vi "CSC_QuadPlannerAdv.vi"(5 "TorqueRelativeWeight":dbl[](array[numeric]), 6 "F range":cluster{"Fmin":dbl, "Fmax":dbl}, 7 "Weight(1e-6)":dbl=1e-06 format="%#_13g", 8 "error in (no error)":errorcluster, 9 "LockedJoint(StartFrom0)":i32[](array[numeric]), 10 "DesireTorque(Nm)":dbl[](array[numeric]) format="%#.4f", 11 "CSC in":refnum<class "CableSerialChain.lvclass">) -> (0 "error out":errorcluster, 1 "Jacobian for Cables":T1 format="%#.3f", 2 "Planned Tension":dbl[](array[numeric]), 3 "CSC out":refnum<class "CableSerialChain.lvclass">, 4 "Solved":bool)   [LabVIEW 2015, in "CableSerialChain.lvclass"]
uses:
  CableSerialChain.lvclass
  <vilib>/Analysis/Matrix/Datatypes/RealMatrix.ctl
  <vilib>/gmath/NumericalOptimization/stopping criteria.ctl
  <vilib>/Analysis/BLAS.llb/LV_Transpose.ctl
  CableSerialChain.lvclass/CableSerialChain.ctl
  <vilib>/Analysis/7linalg.llb/Create Special Real Matrix.vi
  <vilib>/Analysis/Matrix/Numeric/Multiply/Multiply - R,RM.vi
  <vilib>/Analysis/BLAS.llb/dgemv - General Matrix-Vector Product (DBL).vi
  <vilib>/Analysis/BLAS.llb/dgemm - General Matrix-Matrix Product (DBL).vi
  <vilib>/Analysis/Matrix/Numeric/Add/Add - RM,RM.vi
  <vilib>/gmath/NumericalOptimization/Quadratic Programming AS.vi
  <userlib>/_OpenG.lib/error/error.llb/Filter Error Codes (Array)__ogtk.vi
  <vilib>/gmath/NI_Gmath.lvlib
  <vilib>/Analysis/NI_AALPro.lvlib
  <vilib>/Analysis/NI_AALBLAS.lvlib
  <vilib>/Analysis/Matrix/NI_Matrix.lvlib
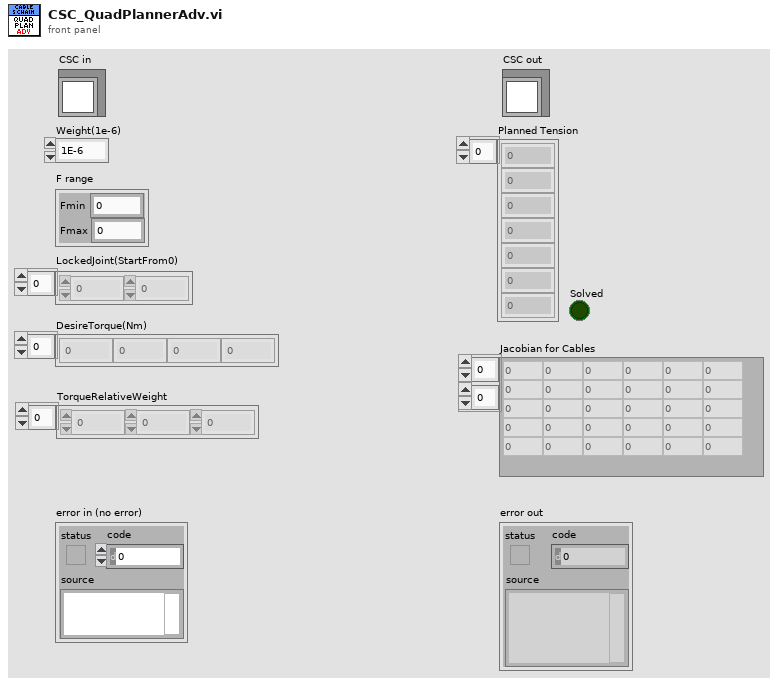
[diagram p1: front panel]
types:
  T1 = typedef "NI_Matrix.lvlib/RealMatrix.ctl" = dbl[][]
  T2 = typedef "NI_Gmath.lvlib/stopping criteria.ctl" = cluster{"function tolerance":dbl, "parameter tolerance":dbl, "max iterations":i32, "max function calls":i32, "gradient tolerance":dbl, "max time (sec)":dbl}
  T3 = typedef "NI_AALBLAS.lvlib/LV_Transpose.ctl" = i32
  T4 = typedef "CableSerialChain.lvclass/Cable.ctl" = cluster{"RoutingPtsInLCS":T5[], "Cable ID":i32, "ActiveSegments":i32[][]}
  T5 = typedef "Bodies.lvclass/PointOnBody.ctl" = cluster{"Coord4":dbl[], "ID":i32}
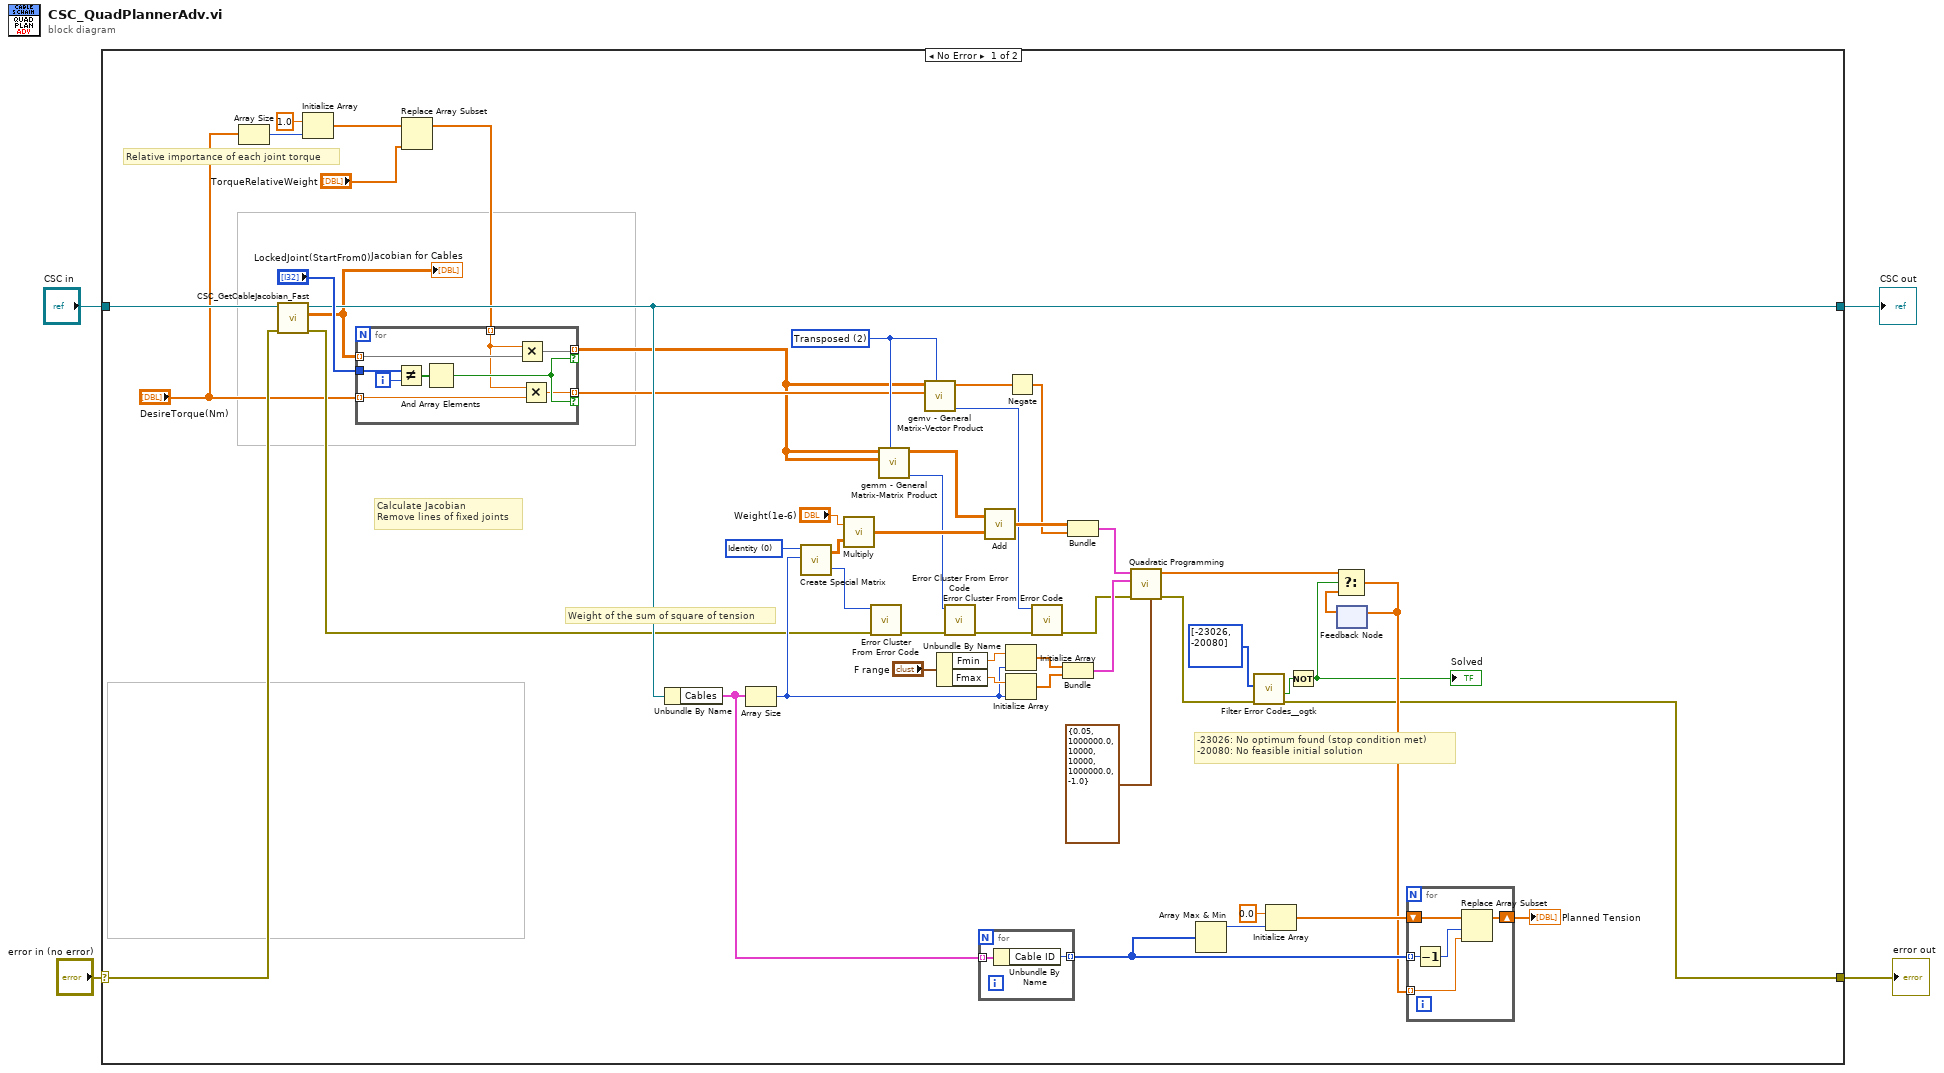
[diagram p0: block diagram]
diagram:
  n1 = case shown="No Error" "error in (no error)" {
    selector: "error in (no error)" -> [w39 w73]
    tunnel: [w15 w73] -> w3
    tunnel: [w38 w74] -> w1
    tunnel: "CSC in" -> [w41 w74]
    frame No Error {
      w30 = T3 2 items=["Direct", "Conjugated & Transposed", "Transposed"] ("operation A")
      w51 = 0 items=["Identity", "Diagonal", "Toeplitz", "Vandermonde", "Companion", "Hankel", "Hadamard", "Wilkinson", "Hilbert", "Inverse Hilbert", "Rosser", "Pascal"] ("matrix type")
      # "-23026: No optimum found (stop condition met)\n-20080: No feasible initial solution"
      # "Weight of the sum of square of tension"
      # "Relative importance of each joint torque"
      # "Calculate Jacobian\nRemove lines of fixed joints"
      n2 = Array Size(array="DesireTorque(Nm)") -> (size(s)=w24:i32)
      n3 = call "CSC_GetCableJacobian_Fast.vi"("error in (no error)"=w39, "C-Alex in"=w41) -> ("error out"=w37:errorcluster, "Jacobian for Cables"=w18:T1, "C-Alex out"=w38:refnum<class "CableSerialChain.lvclass">)  [unwired: 7 in]
      "Jacobian for Cables" <- w18
      n4 = Initialize Array(1.0 ("element"), w24) -> (w22:dbl[])
      n5 = Replace Array Subset(array=w22, new element="TorqueRelativeWeight") -> (w20:dbl[])  [unwired: 1 in]
      n6 = for {
        tunnel: "LockedJoint(StartFrom0)" -> [w71]
        tunnel: w18 -> [w68] mode=indexing
        tunnel: "DesireTorque(Nm)" -> [w64] mode=indexing
        tunnel: [w67] -> w19 mode=indexing if=w69
        tunnel: [w66] -> w29 mode=indexing if=w69
        tunnel: w20 -> [w65] mode=indexing
        i -> [w72]
        n7 = Not Equal?(x=w71, y=w72) -> (x != y?=w70:bool[])
        n8 = And Array Elements(Boolean array=w70) -> (logical AND=w69:bool)
        n9 = Multiply(x=w65, y=w68) -> (x*y=w67:dbl[])
        n10 = Multiply(x=w65, y=w64) -> (x*y=w66:dbl)
      }
      n11 = Unbundle By Name(w38) -> ("Cables"=w40:T4[])
      n12 = Array Size(array=w40) -> (size(s)=w46:i32)
      n13 = call-poly <vilib>:"Create Special Matrix.vi"("matrix type"=w51, "matrix size"=w46) -> ("Special Matrix"=w33:T1, "error"=w49:i32)  [unwired: 3 in]
      n14 = call-poly <vilib>:"Multiply.vi"("Real Matrix A"=w33, "Real Scalar c"="Weight(1e-6)") -> ("c * A"=w26:T1)
      n15 = call <vilib>:"Error Cluster From Error Code.vi"("error in (no error)"=w37, "error code (0)"=w49) -> ("error out"=w6:errorcluster)  [unwired: 7 in]
      n16 = call-poly <vilib>:"gemm - General Matrix-Matrix Product.vi"("operation A"=w30, "B"=w19, "A"=w19) -> ("error"=w9:i32, "dgemm"=w32:T1)  [unwired: 7 in]
      n17 = call-poly <vilib>:"gemv - General Matrix-Vector Product.vi"("operation A"=w30, "x"=w29, "A"=w19) -> ("error"=w8:i32, "dgemv"=w28:dbl[])  [unwired: 7 in]
      n18 = Unbundle By Name("F range") -> ("Fmin"=w55:dbl, "Fmax"=w54:dbl)
      n19 = call <vilib>:"Error Cluster From Error Code.vi"("error in (no error)"=w6, "error code (0)"=w9) -> ("error out"=w7:errorcluster)  [unwired: 7 in]
      n20 = for {
        tunnel: w40 -> [w63] mode=indexing
        tunnel: [w62] -> w44 mode=indexing
        n21 = Unbundle By Name(w63) -> ("Cable ID"=w62:i32)
      }
      n22 = call-poly <vilib>:"Add.vi"("Real Matrix B"=w26, "Real Matrix A"=w32) -> ("A + B"=w31:T1)
      n23 = Initialize Array(w55, w46) -> (w48:dbl[])
      n24 = Initialize Array(w54, w46) -> (w53:dbl[])
      n25 = Negate(x=w28) -> (-x=w27:dbl[])
      n26 = call <vilib>:"Error Cluster From Error Code.vi"("error in (no error)"=w7, "error code (0)"=w8) -> ("error out"=w5:errorcluster)  [unwired: 7 in]
      n27 = Bundle(w48, w53) -> (w52:cluster{dbl[], dbl[]})  [unwired: 1 in]
      n28 = Bundle("A + B"=w31, w27) -> (w50:cluster{"A + B":T1, dbl[]})  [unwired: 1 in]
      n29 = call-poly <vilib>:"Quadratic Programming.vi"("stopping criteria"=T2 {"function tolerance"=0.05, "parameter tolerance"=1000000.0, "max iterations"=10000, "max function calls"=10000, "gradient tolerance"=1000000.0, "max time (sec)"=-1.0}, "error in (no error)"=w5, "parameter bounds"=w52, "objective function"=w50) -> ("error out"=w16:errorcluster, "minimum"=w11:dbl[])  [unwired: 4 in, 2 out]
      n30 = Array Max & Min(array=w44) -> (max value=w43:i32)  [unwired: 3 out]
      n31 = call-poly <userlib>:"Filter Error Codes__ogtk.vi"("Error In"=w16, "Error Codes to Filter"=i32[] [-23026, -20080]) -> ("Error Out"=w15:errorcluster, "Error Filtered?"=w14:bool)  [unwired: 7 in, 1 out]
      n32 = Initialize Array(0.0 ("element"), w43) -> (w42:dbl[])
      n33 = Not(x=w14) -> (.not. x?=w12:bool)
      "Solved" <- w12
      n34 = feedback #1() -> (w10:dbl[])  [unwired: 1 in]
      n35 = Select(t=w11, s=w12, f=w10) -> (s? t:f=w36:dbl[])
      n36 = feedback-in #1(w36) -> ()
      n37 = for {
        tunnel: w44 -> [w61] mode=indexing
        shift-right: [w59] -> w17
        shift-left: w42 -> [w58]
        tunnel: w36 -> [w57] mode=indexing
        n38 = Decrement(x=w61) -> (x-1=w60:i32)
        n39 = Replace Array Subset(array=w58, new element=w57, index=w60) -> (w59:dbl[])
      }
      "Planned Tension" <- w17
    }
    frame Error {
    }
  }
  "error out" <- w3
  "CSC out" <- w1
